vi "Read VISA.vi"(7 "Opciones":T1(ring), 8 "error in (no error)":errorcluster, 9 "Write":string, 10 "baud rate (9600)":u32=115200, 11 "VISA com port":refnum<visa-resource-name>) -> (0 "error out":errorcluster, 2 "Read":string, 3 "VISA com port 2":refnum<visa-resource-name>)   [LabVIEW 2020]
uses:
  <vilib>/Instr/_visa.llb/VISA Configure Serial Port (Instr).vi
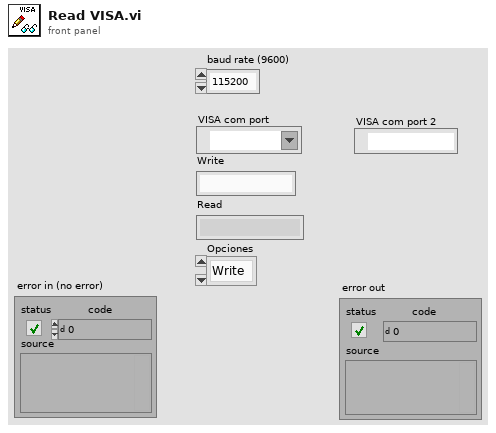
[diagram p1: front panel]
types:
  T1 = enum16{"Write", "Read", "Config", "Reset", "Close"}
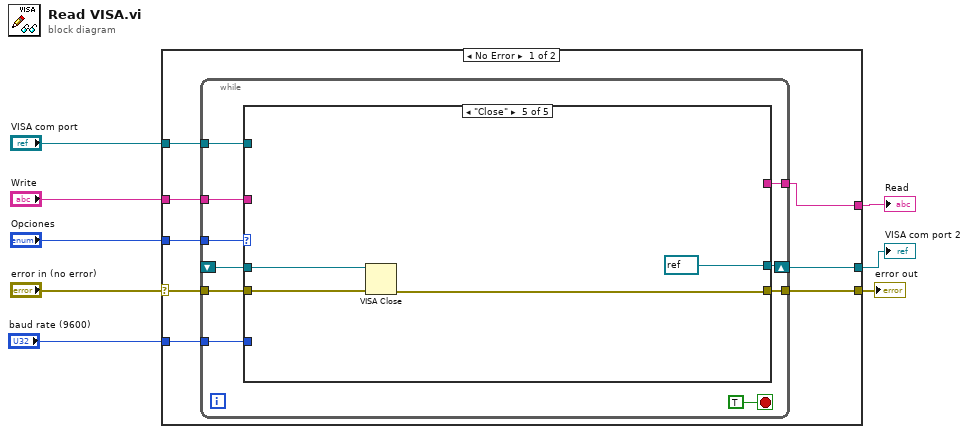
[diagram p0: block diagram]
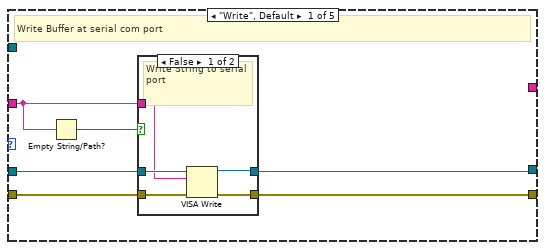
[diagram p2: hidden frame]
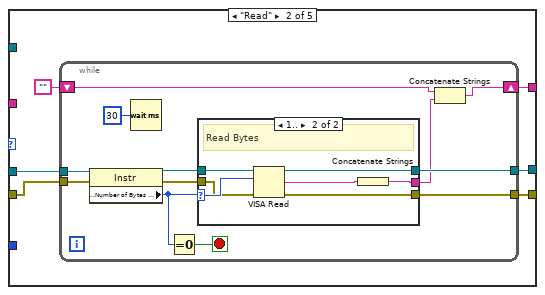
[diagram p4: hidden frame]
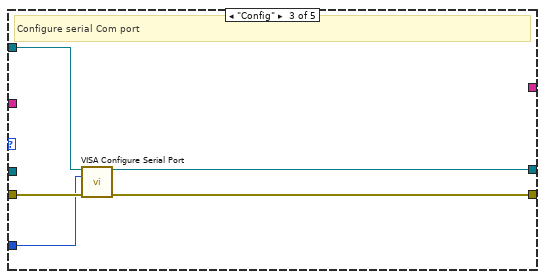
[diagram p6: hidden frame]
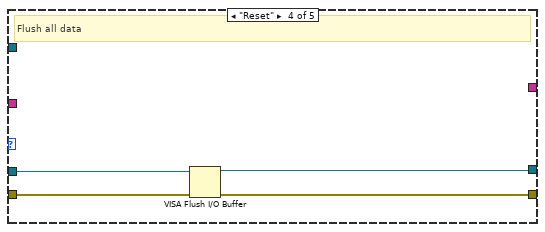
[diagram p7: hidden frame]
diagram:
  n1 = case shown="No Error" "error in (no error)" {
    selector: "error in (no error)" -> [w15 w80]
    tunnel: [w14 w80] -> w7
    tunnel: "Opciones" -> [w16 _]
    tunnel: "VISA com port" -> [w13 _]
    tunnel: "Write" -> [w12 _]
    tunnel: [w11 _] -> w3
    tunnel: "baud rate (9600)" -> [w10 _]
    tunnel: [w9 _] -> w1
    frame No Error {
      n2 = while {
        tunnel: w16 -> [w25]
        tunnel: w15 -> [w24]
        tunnel: [w23] -> w14
        tunnel: w13 -> [w22]
        shift-right: [w21] -> w9
        shift-left: _ -> [w20]
        tunnel: w12 -> [w19]
        tunnel: [w18] -> w11
        tunnel: w10 -> [w17]
        stop <- TRUE stop-if-true
        n3 = case shown="\"Close\"" w25 {
          tunnel: w24 -> [w32 w44 w71 w75 w79]
          tunnel: [w31 w43 w68 w74 w78] -> w23
          tunnel: w22 -> [_ _ w70 _ _]
          tunnel: [w27 w42 w69 w72 refnum<visa-resource-name> refnum ("VISA resource name out")] -> w21
          tunnel: w20 -> [w30 w45 _ w73 w77]
          tunnel: w19 -> [w29 _ _ _ _]
          tunnel: [_ w41 _ _ _] -> w18
          tunnel: w17 -> [_ _ w67 _ _]
          frame "Write", Default {
            # "Write Buffer at serial com port"
            n4 = Empty String/Path?(string/path=w29) -> (empty?=w28:bool)
            n5 = case shown="False" w28 {
              tunnel: w32 -> [w37 w38]
              tunnel: [w36 w38] -> w31
              tunnel: w30 -> [w35 w39]
              tunnel: w29 -> [w34 _]
              tunnel: [w33 w39] -> w27
              frame False {
                # "Write String to serial port"
                n6 = VISA Write(VISA resource name=w35, write buffer=w34, error in (no error)=w37) -> (VISA resource name out=w33:refnum<visa-resource-name>, error out=w36:errorcluster)  [unwired: 1 out]
              }
              frame True {
              }
            }
          }
          frame "Read" {
            n7 = while {
              tunnel: w45 -> [w57]
              tunnel: w44 -> [w56]
              tunnel: [w53] -> w43
              tunnel: [w52] -> w42
              shift-right: [w47] -> w41
              shift-left: "" -> [w46]
              stop <- w49 stop-if-true
              n8 = property class="Instr"(reference=w57, error in=w56) -> (reference out=w55:refnum<visa-resource-name>, error out=w54:errorcluster, "Serial Settings:Number of Bytes at Serial Port"=w50:u32)
              n9 = Wait (ms)(milliseconds to wait=u32 30) -> ()  [unwired: 1 out]
              n10 = Equal To 0?(x=w50) -> (x = 0?=w49:bool)
              n11 = case shown="1.." w50 {
                selector: w50 -> [_ w65]
                tunnel: w55 -> [w59 w66]
                tunnel: w54 -> [w58 w62]
                tunnel: [w58 w64] -> w53
                tunnel: [w59 w63] -> w52
                tunnel: [_ w60] -> w48
                frame 0, Default {
                }
                frame 1.. {
                  # "Read Bytes"
                  n12 = VISA Read(VISA resource name=w66, byte count=w65, error in (no error)=w62) -> (VISA resource name out=w63:refnum<visa-resource-name>, read buffer=w61:string, error out=w64:errorcluster)  [unwired: 1 out]
                  n13 = Concatenate Strings(w61) -> (w60:string)
                }
              }
              n14 = Concatenate Strings(w46, w48) -> (w47:string)
            }
          }
          frame "Config" {
            # "Configure serial Com port"
            n15 = call-poly "VISA Configure Serial Port"("VISA resource name"=w70, "baud rate (9600)"=w67, "error in (no error)"=w71) -> ("VISA resource name out"=w69:refnum<visa-resource-name>, "error out"=w68:errorcluster)  [unwired: 11 in]
          }
          frame "Reset" {
            # "Flush all data"
            n16 = VISA Flush I/O Buffer(VISA resource name=w73, error in (no error)=w75) -> (VISA resource name out=w72:refnum<visa-resource-name>, error out=w74:errorcluster)  [unwired: 1 in]
          }
          frame "Close" {
            n17 = VISA Close(VISA resource name=w77, error in (no error)=w79) -> (error out=w78:errorcluster)
          }
        }
      }
    }
    frame Error {
    }
  }
  "error out" <- w7
  "Read" <- w3
  "VISA com port 2" <- w1
